vi "Read Number of Channel.vi"(11 "E3631A in":refnum<class "E3631A.lvclass">) -> (2 "Number of Channel":dbl, 3 "E3631A out":refnum<class "E3631A.lvclass">)   [LabVIEW 2020, in "E3631A.lvclass"]
uses:
  E3631A.lvclass
  E3631A.lvclass/E3631A.ctl
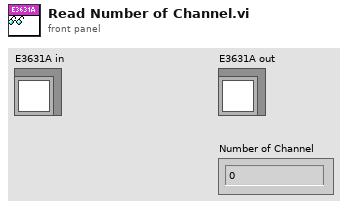
[diagram p1: front panel]
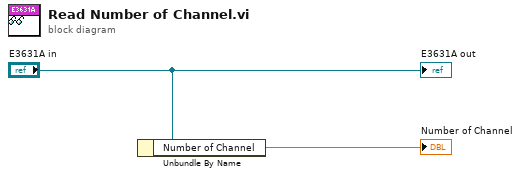
[diagram p0: block diagram]
diagram:
  n1 = Unbundle By Name("E3631A in") -> ("Number of Channel"=→"Number of Channel":dbl)
  "E3631A out" <- "E3631A in"
